vi "sub_apt_setjoystick.vi"   [LabVIEW 2015]
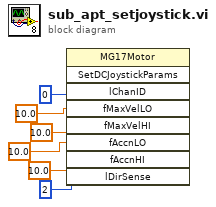
[diagram p0: block diagram]
diagram:
  n1 = invoke class="MG17Motor" method="SetDCJoystickParams"("lChanID"=0, "fMaxVelLO"=sgl 10.0, "fMaxVelHI"=sgl 10.0, "fAccnLO"=sgl 10.0, "fAccnHI"=sgl 10.0, "lDirSense"=2) -> ()  [unwired: 3 in, 9 out]
